vi "HV_VSet_Multi.vi"(8 "Voltage":string[](array[string]), 11 "Channel":string[](array[string])) -> (3 "Output":string[](array[string]))   [LabVIEW 2018]
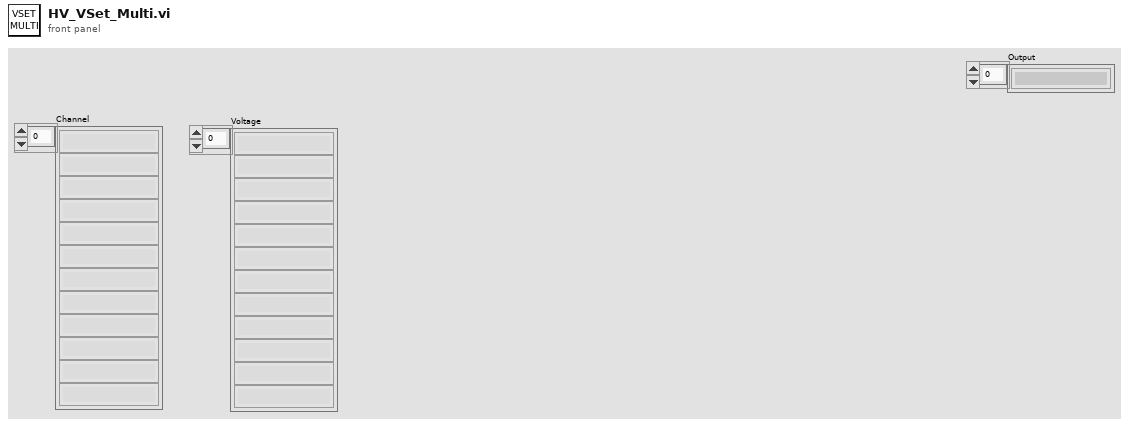
[diagram p1: front panel]
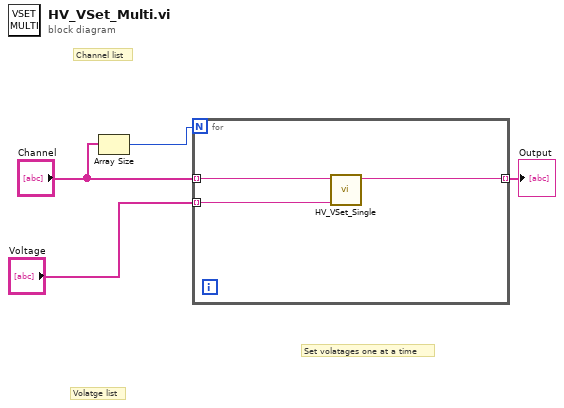
[diagram p0: block diagram]
diagram:
  # "Set volatages one at a time"
  # "Volatge list"
  # "Channel list"
  n1 = Array Size(array="Channel") -> (size(s)=w2:i32)
  n2 = for {
    N: w2 -> [_]
    tunnel: "Channel" -> [w7] mode=indexing
    tunnel: "Voltage" -> [w6] mode=indexing
    tunnel: [w5] -> w1 mode=indexing
    n3 = call "HV_VSet_Single.vi"("Voltage"=w6, "Channel"=w7) -> ("standard output"=w5:string)  [unwired: 9 in]
  }
  "Output" <- w1
